vi "PicoScope5000aGetRapidBlock.vi"(0 "error in":errorcluster, 1 "enabled array":i16[](array[numeric]), 7 "handle in":i16, 9 "Buffer and Transfer Settings":T1={"startIndex"=0, "Samples"=1000, "Down Sample Ratio"=1, "Down-Sample Mode"=1} {"Down-Sample Mode" items=["None"=0, "Aggregate"=1, "Decimate"=2, "Average"=4]; "Down Sample Ratio" step=1; "Samples" format="%_6p"}, 11 "Rapid Block Acquisition Settings":T2={"preTriggerSamples"=0, "postTriggerSamples"=1000, "timebase"=2, "Four Channel Device"=FALSE, "Number of Captures"=1}) -> (2 "Channel A Buffer":i16[][](array[numeric]), 3 "Channel B Buffer":i16[][](array[numeric]), 4 "error out":errorcluster, 6 "handle out":i16, 8 "Port 0":i16[][](array[numeric]), 10 "Port 1":i16[][](array[numeric]), 12 "noOfSamples":u32[](array[numeric]), 13 "Channel C Buffer":i16[][](array[numeric]), 14 "Channel D Buffer":i16[][](array[numeric]))   [LabVIEW 2010]
doc: "This VI gets a set of blocks captured using rapid block mode. It outputs two-dimensional arrays for each channel that contain data from all the requested captures."
uses:
  ps5000a.dll
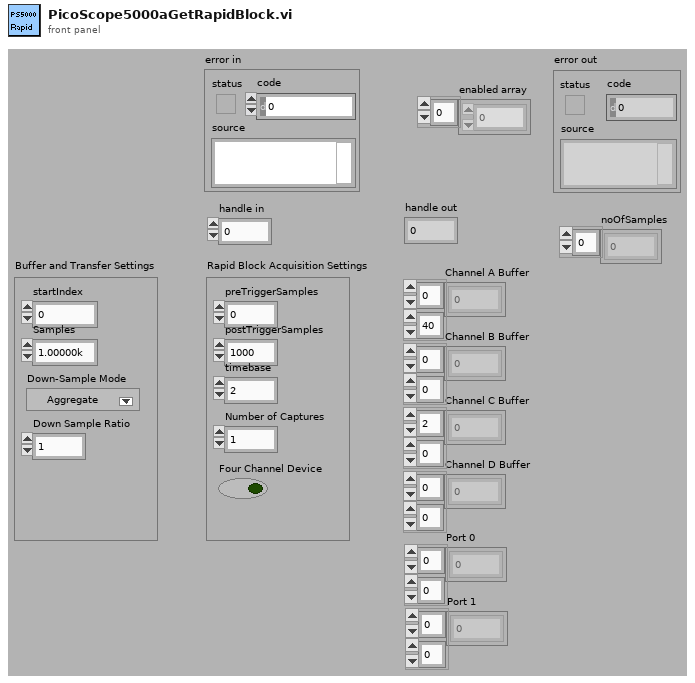
[diagram p1: front panel]
types:
  T1 = cluster{"startIndex":u64, "Samples":u64, "Down Sample Ratio":u64, "Down-Sample Mode":u32}
  T2 = cluster{"preTriggerSamples":i32, "postTriggerSamples":i32, "timebase":u32, "Four Channel Device":bool, "Number of Captures":u32}
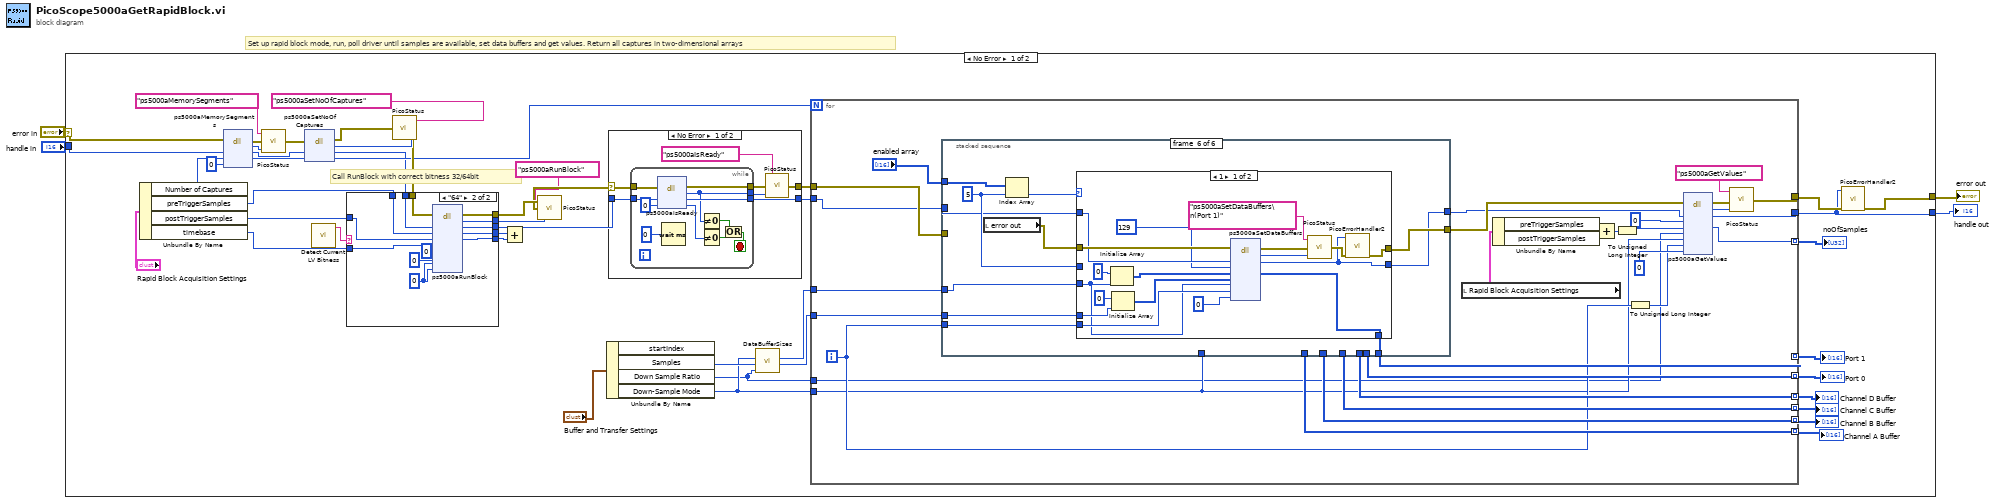
[diagram p0: block diagram]
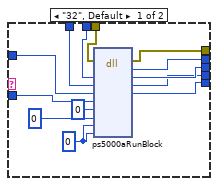
[diagram p2: hidden frame]
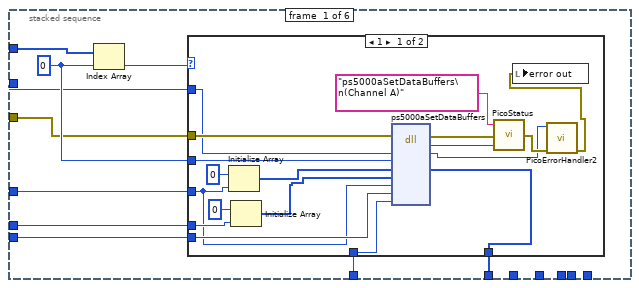
[diagram p3: hidden frame]
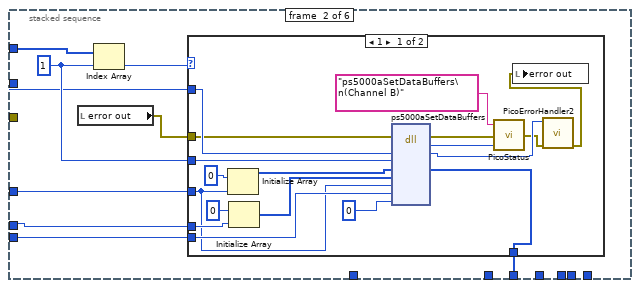
[diagram p5: hidden frame]
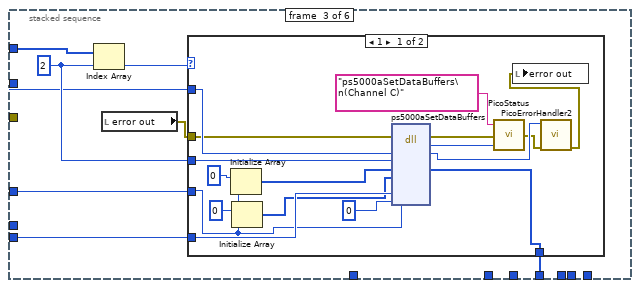
[diagram p7: hidden frame]
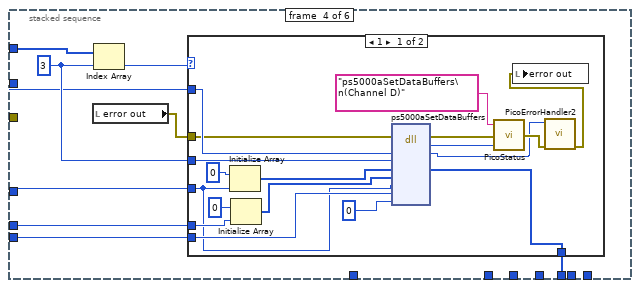
[diagram p9: hidden frame]
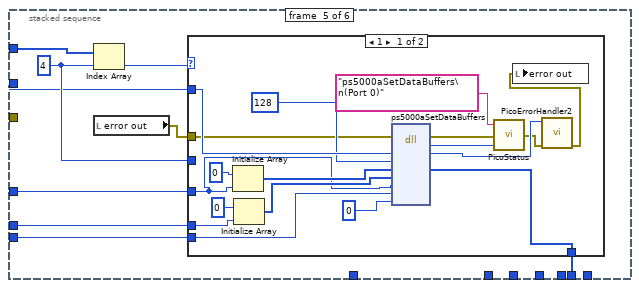
[diagram p11: hidden frame]
diagram:
  # "Set up rapid block mode, run, poll driver until samples are available, set data buffers and get values. Return all captures in two-dimensional arrays"
  n1 = case shown="No Error" "error in" {
    selector: "error in" -> [w42 w293]
    tunnel: [w22 w293] -> w1
    tunnel: "handle in" -> [w41 w292]
    tunnel: [w19 w292] -> w2
    frame No Error {
      # "Call RunBlock with correct bitness 32/64bit"
      n2 = Unbundle By Name("Rapid Block Acquisition Settings") -> ("Number of Captures"=w37:u32, "preTriggerSamples"=w15:i32, "postTriggerSamples"=w14:i32, "timebase"=w13:u32)
      n3 = dll-call lib="ps5000a.dll" fn="ps5000aMemorySegments" ("ps3000.dll:_ps3000_open_unit@0")(error in=w42, "handle"=w41, "nSegments"=w37, "nMaxSamples"=0) -> (error out=w39:errorcluster, "PICO_STATUS"=w40:u32, "handle"=w34:i16, "nSegments"=w35:u32)  [unwired: 3 in, 1 out]
      n4 = call "PicoStatus.vi"("PICO STATUS"=w40, "error in"=w39, "source"="ps5000aMemorySegments") -> ("error out"=w33:errorcluster)
      n5 = dll-call lib="ps5000a.dll" fn="ps5000aSetNoOfCaptures" ("ps3000.dll:_ps3000_open_unit@0")(error in=w33, "handle"=w34, "nCaptures"=w35) -> (error out=w31:errorcluster, "PICO_STATUS"=w32:u32, "handle"=w16:i16, "nCaptures"=w28:u32)  [unwired: 2 in, 1 out]
      n6 = call "Detect Current LV Bitness.vi"() -> ("bitness"=w17:string)  [unwired: 11 in]
      n7 = call "PicoStatus.vi"("PICO STATUS"=w32, "error in"=w31, "source"="ps5000aSetNoOfCaptures") -> ("error out"=w29:errorcluster)
      n8 = case shown="\"64\"" w17 {
        tunnel: [w55 w76] -> w50
        tunnel: [w56 w75] -> w46
        tunnel: [w57 w74] -> w45
        tunnel: w29 -> [w63 w73]
        tunnel: w16 -> [w62 w72]
        tunnel: w15 -> [w61 w71]
        tunnel: w14 -> [w60 w70]
        tunnel: w13 -> [w59 w68]
        tunnel: [w53 w67] -> w12
        tunnel: [w54 w66] -> w11
        frame "32", Default {
          w51 = u32 0 ("pParameter")
          n9 = dll-call lib="ps5000a.dll" fn="ps5000aRunBlock" ("ps3000.dll:_ps3000_open_unit@0")(error in=w63, "handle"=w62, "preTriggerSamples"=w61, "postTriggerSamples"=w60, "timebase"=w59, "timeindisposedMs"=0, "segmentIndex"=u32 0, "lpReady"=w51, "pParameter"=w51) -> (error out=w57:errorcluster, "PICO_STATUS"=w56:u32, "handle"=w55:i16, "preTriggerSamples"=w54:i32, "postTriggerSamples"=w53:i32)  [unwired: 7 in, 1 out]
        }
        frame "64" {
          w64 = u64 0 ("pParameter")
          n10 = dll-call lib="ps5000a.dll" fn="ps5000aRunBlock" ("ps3000.dll:_ps3000_open_unit@0")(error in=w73, "handle"=w72, "preTriggerSamples"=w71, "postTriggerSamples"=w70, "timebase"=w68, "timeindisposedMs"=0, "segmentIndex"=u32 0, "lpReady"=w64, "pParameter"=w64) -> (error out=w74:errorcluster, "PICO_STATUS"=w75:u32, "handle"=w76:i16, "preTriggerSamples"=w66:i32, "postTriggerSamples"=w67:i32)  [unwired: 7 in, 1 out]
        }
      }
      n11 = Add(x=w11, y=w12) -> ()  [unwired: 1 out]
      n12 = call "PicoStatus.vi"("PICO STATUS"=w46, "error in"=w45, "source"="ps5000aRunBlock") -> ("error out"=w44:errorcluster)
      n13 = Unbundle By Name("Buffer and Transfer Settings") -> ("Samples"=w9:u64, "Down Sample Ratio"=w5:u64, "Down-Sample Mode"=w8:u32)  [unwired: 1 out]
      n14 = case shown="No Error" w44 {
        selector: w44 -> [w276 w290]
        tunnel: w50 -> [w278 w291]
        tunnel: [w277 w291] -> w49
        tunnel: [w275 w290] -> w48
        frame No Error {
          n15 = while {
            tunnel: [w289] -> w277
            tunnel: w278 -> [w288]
            tunnel: [w283] -> w273
            tunnel: w276 -> [w282]
            tunnel: [w281] -> w274
            stop <- w287 stop-if-true
            n16 = dll-call lib="ps5000a.dll" fn="ps5000aIsReady" ("ps3000.dll:_ps3000_open_unit@0")(error in=w282, "handle"=w288, "ready"=i16 0) -> (error out=w281:errorcluster, "PICO_STATUS"=w283:u32, "handle"=w289:i16, "ready"=w284:i16)  [unwired: 2 in, 1 out]
            n17 = Wait (ms)(milliseconds to wait=i16 0 ("ready")) -> ()  [unwired: 1 out]
            n18 = Not Equal To 0?(x=w283) -> (x != 0?=w285:bool)
            n19 = Not Equal To 0?(x=w284) -> (x != 0?=w286:bool)
            n20 = Or(x=w285, y=w286) -> (x .or. y?=w287:bool)
          }
          n21 = call "PicoStatus.vi"("PICO STATUS"=w273, "error in"=w274, "source"="ps5000aIsReady") -> ("error out"=w275:errorcluster)
        }
        frame Error {
        }
      }
      n22 = call "DataBufferSizes.vi"("Down Sample Ratio"=w5, "Number of Samples"=w9, "Down-Sample Mode"=w8) -> ("min Buffer Size"=w6:i32, "Max Buffer Size"=w7:i32)  [unwired: 7 in]
      n23 = for {
        N: w28 -> [_]
        tunnel: w49 -> [w92]
        tunnel: w48 -> [w94]
        tunnel: [w86] -> w27 mode=indexing
        tunnel: [w87] -> w26 mode=indexing
        tunnel: [w88] -> w25 mode=indexing
        tunnel: [w89] -> w24 mode=indexing
        tunnel: [w98] -> w19
        tunnel: [w97] -> w23
        tunnel: [w85] -> w21 mode=indexing
        tunnel: [w84] -> w20 mode=indexing
        tunnel: [w81] -> w18 mode=indexing
        tunnel: w8 -> [w78]
        tunnel: w7 -> [w80]
        tunnel: w6 -> [w79]
        tunnel: w5 -> [w77]
        i -> [w82]
        n24 = stacked-sequence {
          tunnel: "enabled array" -> [w115 w142 w168 w194 w221 w250]
          tunnel: w94 -> [w113 _ _ _ _ _]
          tunnel: w92 -> [w112 w140 w166 w192 w219 w248]
          tunnel: [w111 _ _ _ _ _] -> w89
          tunnel: [_ _ _ _ _ w246] -> w95
          tunnel: [_ _ _ _ _ w245] -> w93
          tunnel: w82 -> [w107 w139 w165 w191 w218 w247]
          tunnel: [_ w138 _ _ _ _] -> w88
          tunnel: [_ _ w164 _ _ _] -> w87
          tunnel: [_ _ _ w190 _ _] -> w86
          tunnel: [_ _ _ _ w217 _] -> w85
          tunnel: [_ _ _ _ _ w243] -> w84
          tunnel: w78 -> [w110 _ _ _ _ _]
          tunnel: w80 -> [w109 w137 w163 w189 w216 w242]
          tunnel: w79 -> [w108 w136 _ w188 w215 w241]
          frame #0 {
            w116 = 0 ("dimension size")
            n25 = Index Array(array=w115, index=w116) -> (element=w114:i16)
            n26 = case shown="1" w114 {
              tunnel: w116 -> [w131 _]
              tunnel: w113 -> [w133 _]
              tunnel: w112 -> [w132 _]
              tunnel: [w130 _] -> w111
              tunnel: w107 -> [w129 _]
              tunnel: w110 -> [w123 _]
              tunnel: w109 -> [w117 _]
              tunnel: w108 -> [w118 _]
              frame 1 {
                n27 = Initialize Array(i16 0 ("element"), w117) -> (w120:i16[])
                n28 = Initialize Array(i16 0 ("element"), w118) -> (w119:i16[])
                n29 = dll-call lib="ps5000a.dll" fn="ps5000aSetDataBuffers" ("ps3000.dll:_ps3000_open_unit@0")(error in=w133, "handle"=w132, "channel"=w131, "bufferMax"=w120, "bufferMin"=w119, "bufferLth"=w117, "segmentIndex"=w129, "downSampleRatioMode"=w123) -> (error out=w128:errorcluster, "PICO_STATUS"=w125:u32, "handle"=w124:i16, "bufferMax"=w130:i16[])  [unwired: 7 in, 1 out]
                n30 = call "PicoStatus.vi"("PICO STATUS"=w125, "error in"=w128, "source"="ps5000aSetDataBuffers\n(Channel A)") -> ("error out"=w127:errorcluster)
                n31 = call "PicoErrorHandler2.vi"("error in (no error)"=w127, "handle In"=w124) -> ("error out"=w126:errorcluster)  [unwired: 9 in]
                n32 = local write "error out"(w126) -> ()
              }
              frame 0, Default {
              }
            }
          }
          frame #1 {
            w143 = 1 ("dimension size")
            n33 = local read "error out"() -> (w135:errorcluster)
            n34 = Index Array(array=w142, index=w143) -> (element=w141:i16)
            n35 = case shown="1" w141 {
              tunnel: w143 -> [w159 _]
              tunnel: w140 -> [w160 _]
              tunnel: [w158 _] -> w138
              tunnel: w139 -> [w157 _]
              tunnel: w137 -> [w145 _]
              tunnel: w136 -> [w147 _]
              tunnel: w135 -> [w144 _]
              frame 1 {
                n36 = Initialize Array(i16 0 ("element"), w145) -> (w148:i16[])
                n37 = Initialize Array(i16 0 ("element"), w147) -> (w146:i16[])
                n38 = dll-call lib="ps5000a.dll" fn="ps5000aSetDataBuffers" ("ps3000.dll:_ps3000_open_unit@0")(error in=w144, "handle"=w160, "channel"=w159, "bufferMax"=w148, "bufferMin"=w146, "bufferLth"=w145, "segmentIndex"=w157, "downSampleRatioMode"=u32 0 ("segmentIndex")) -> (error out=w155:errorcluster, "PICO_STATUS"=w154:u32, "handle"=w152:i16, "bufferMax"=w158:i16[])  [unwired: 7 in, 1 out]
                n39 = call "PicoStatus.vi"("PICO STATUS"=w154, "error in"=w155, "source"="ps5000aSetDataBuffers\n(Channel B)") -> ("error out"=w151:errorcluster)
                n40 = call "PicoErrorHandler2.vi"("error in (no error)"=w151, "handle In"=w152) -> ("error out"=w153:errorcluster)  [unwired: 9 in]
                n41 = local write "error out"(w153) -> ()
              }
              frame 0, Default {
              }
            }
          }
          frame #2 {
            w169 = 2 ("dimension size")
            n42 = Index Array(array=w168, index=w169) -> (element=w167:i16)
            n43 = local read "error out"() -> (w162:errorcluster)
            n44 = case shown="1" w167 {
              tunnel: w169 -> [w184 _]
              tunnel: w166 -> [w185 _]
              tunnel: [w183 _] -> w164
              tunnel: w165 -> [w182 _]
              tunnel: w163 -> [w171 _]
              tunnel: w162 -> [w170 _]
              frame 1 {
                n45 = Initialize Array(i16 0 ("element"), w171) -> (w173:i16[])
                n46 = Initialize Array(i16 0 ("element")) -> (w172:i16[])  [unwired: 1 in]
                n47 = dll-call lib="ps5000a.dll" fn="ps5000aSetDataBuffers" ("ps3000.dll:_ps3000_open_unit@0")(error in=w170, "handle"=w185, "channel"=w184, "bufferMax"=w173, "bufferMin"=w172, "bufferLth"=w171, "segmentIndex"=w182, "downSampleRatioMode"=u32 0 ("segmentIndex")) -> (error out=w180:errorcluster, "PICO_STATUS"=w179:u32, "handle"=w178:i16, "bufferMax"=w183:i16[])  [unwired: 7 in, 1 out]
                n48 = call "PicoStatus.vi"("PICO STATUS"=w179, "error in"=w180, "source"="ps5000aSetDataBuffers\n(Channel C)") -> ("error out"=w177:errorcluster)
                n49 = call "PicoErrorHandler2.vi"("error in (no error)"=w177, "handle In"=w178) -> ("error out"=w176:errorcluster)  [unwired: 9 in]
                n50 = local write "error out"(w176) -> ()
              }
              frame 0, Default {
              }
            }
          }
          frame #3 {
            w195 = 3 ("dimension size")
            n51 = local read "error out"() -> (w187:errorcluster)
            n52 = Index Array(array=w194, index=w195) -> (element=w193:i16)
            n53 = case shown="1" w193 {
              tunnel: w195 -> [w211 _]
              tunnel: w192 -> [w212 _]
              tunnel: [w210 _] -> w190
              tunnel: w191 -> [w209 _]
              tunnel: w189 -> [w197 _]
              tunnel: w188 -> [w200 _]
              tunnel: w187 -> [w196 _]
              frame 1 {
                n54 = Initialize Array(i16 0 ("element"), w197) -> (w199:i16[])
                n55 = Initialize Array(i16 0 ("element"), w200) -> (w198:i16[])
                n56 = dll-call lib="ps5000a.dll" fn="ps5000aSetDataBuffers" ("ps3000.dll:_ps3000_open_unit@0")(error in=w196, "handle"=w212, "channel"=w211, "bufferMax"=w199, "bufferMin"=w198, "bufferLth"=w197, "segmentIndex"=w209, "downSampleRatioMode"=u32 0 ("segmentIndex")) -> (error out=w207:errorcluster, "PICO_STATUS"=w206:u32, "handle"=w203:i16, "bufferMax"=w210:i16[])  [unwired: 7 in, 1 out]
                n57 = call "PicoStatus.vi"("PICO STATUS"=w206, "error in"=w207, "source"="ps5000aSetDataBuffers\n(Channel D)") -> ("error out"=w204:errorcluster)
                n58 = call "PicoErrorHandler2.vi"("error in (no error)"=w204, "handle In"=w203) -> ("error out"=w205:errorcluster)  [unwired: 9 in]
                n59 = local write "error out"(w205) -> ()
              }
              frame 0, Default {
              }
            }
          }
          frame #4 {
            w222 = 4 ("dimension size")
            n60 = Index Array(array=w221, index=w222) -> (element=w220:i16)
            n61 = local read "error out"() -> (w214:errorcluster)
            n62 = case shown="1" w220 {
              tunnel: w222 -> [_ _]
              tunnel: w219 -> [w239 _]
              tunnel: [w238 _] -> w217
              tunnel: w218 -> [w237 _]
              tunnel: w216 -> [w224 _]
              tunnel: w215 -> [w227 _]
              tunnel: w214 -> [w223 _]
              frame 1 {
                n63 = Initialize Array(i16 0 ("element"), w224) -> (w226:i16[])
                n64 = Initialize Array(i16 0 ("element"), w227) -> (w225:i16[])
                n65 = dll-call lib="ps5000a.dll" fn="ps5000aSetDataBuffers" ("ps3000.dll:_ps3000_open_unit@0")(error in=w223, "handle"=w239, "channel"=u32 128, "bufferMax"=w226, "bufferMin"=w225, "bufferLth"=w224, "segmentIndex"=w237, "downSampleRatioMode"=u32 0 ("segmentIndex")) -> (error out=w235:errorcluster, "PICO_STATUS"=w234:u32, "handle"=w232:i16, "bufferMax"=w238:i16[])  [unwired: 7 in, 1 out]
                n66 = call "PicoStatus.vi"("PICO STATUS"=w234, "error in"=w235, "source"="ps5000aSetDataBuffers\n(Port 0)") -> ("error out"=w231:errorcluster)
                n67 = call "PicoErrorHandler2.vi"("error in (no error)"=w231, "handle In"=w232) -> ("error out"=w230:errorcluster)  [unwired: 9 in]
                n68 = local write "error out"(w230) -> ()
              }
              frame 0, Default {
              }
            }
          }
          frame #5 {
            w251 = 5 ("dimension size")
            n69 = local read "error out"() -> (w244:errorcluster)
            n70 = Index Array(array=w250, index=w251) -> (element=w249:i16)
            n71 = case shown="1" w249 {
              tunnel: w251 -> [_ _]
              tunnel: w244 -> [w268 w270]
              tunnel: w248 -> [w267 w271]
              tunnel: [w266 _] -> w243
              tunnel: w247 -> [w265 _]
              tunnel: [w260 w270] -> w246
              tunnel: [w258 w271] -> w245
              tunnel: w242 -> [w252 _]
              tunnel: w241 -> [w255 _]
              frame 1 {
                n72 = Initialize Array(i16 0 ("element"), w252) -> (w254:i16[])
                n73 = Initialize Array(i16 0 ("element"), w255) -> (w253:i16[])
                n74 = dll-call lib="ps5000a.dll" fn="ps5000aSetDataBuffers" ("ps3000.dll:_ps3000_open_unit@0")(error in=w268, "handle"=w267, "channel"=u32 129, "bufferMax"=w254, "bufferMin"=w253, "bufferLth"=w252, "segmentIndex"=w265, "downSampleRatioMode"=u32 0 ("segmentIndex")) -> (error out=w263:errorcluster, "PICO_STATUS"=w262:u32, "handle"=w258:i16, "bufferMax"=w266:i16[])  [unwired: 7 in, 1 out]
                n75 = call "PicoStatus.vi"("PICO STATUS"=w262, "error in"=w263, "source"="ps5000aSetDataBuffers\n(Port 1)") -> ("error out"=w259:errorcluster)
                n76 = call "PicoErrorHandler2.vi"("error in (no error)"=w259, "handle In"=w258) -> ("error out"=w260:errorcluster)  [unwired: 9 in]
              }
              frame 0, Default {
              }
            }
          }
        }
        n77 = local read "Rapid Block Acquisition Settings"() -> (w103:T2)
        n78 = Unbundle By Name(w103) -> ("preTriggerSamples"=w105:i32, "postTriggerSamples"=w104:i32)
        n79 = Add(x=w105, y=w104) -> (x+y=w106:i32)
        n80 = To Unsigned Long Integer(number=w106) -> (unsigned 32bit integer=w96:u32)
        n81 = To Unsigned Long Integer(number=w82) -> (unsigned 32bit integer=w83:u32)
        n82 = dll-call lib="ps5000a.dll" fn="ps5000aGetValues" ("ps3000.dll:_ps3000_open_unit@0")(error in=w95, "handle"=w93, "startIndex"=u32 0, "noOfSamples"=w96, "downSampleRatio"=w77, "downSampleRatioMode"=w78, "segmentIndex"=w83, "overflow"=i16 0) -> (error out=w100:errorcluster, "PICO_STATUS"=w99:u32, "handle"=w98:i16, "noOfSamples"=w81:u32)  [unwired: 7 in, 1 out]
        n83 = call "PicoStatus.vi"("PICO STATUS"=w99, "error in"=w100, "source"="ps5000aGetValues") -> ("error out"=w97:errorcluster)
      }
      "Channel D Buffer" <- w27
      "Channel C Buffer" <- w26
      "Channel B Buffer" <- w25
      "Channel A Buffer" <- w24
      "Port 0" <- w21
      "Port 1" <- w20
      "noOfSamples" <- w18
      n84 = call "PicoErrorHandler2.vi"("error in (no error)"=w23, "handle In"=w19) -> ("error out"=w22:errorcluster)  [unwired: 9 in]
    }
    frame Error {
    }
  }
  "handle out" <- w2
  "error out" <- w1
